vi "Set Point.vi"(8 "error in (no error)":errorcluster, 9 "Output #":i32=1, 10 "Set point":dbl, 11 "Cryo-Con Driver in":refnum<class "Cryo-Con Driver.lvclass">) -> (0 "error out":errorcluster, 3 "Cryo-Con Driver out":refnum<class "Cryo-Con Driver.lvclass">)   [LabVIEW 2021, in "Cryo-Con Driver.lvclass"]
uses:
  Cryo-Con Driver.lvclass
  C:/GitHub/NHMFL_Core/Libraries/Instruments/VISA Instrument/VISA Instrument.lvclass
  VISA Instrument/VISA Instrument.lvclass/VISA Instrument.ctl
  VISA Instrument/Read VISA resource.vi
  VISA Instrument/Write VISA resource.vi
  Cryo-Con Driver.lvclass/Cryo-Con Driver.ctl
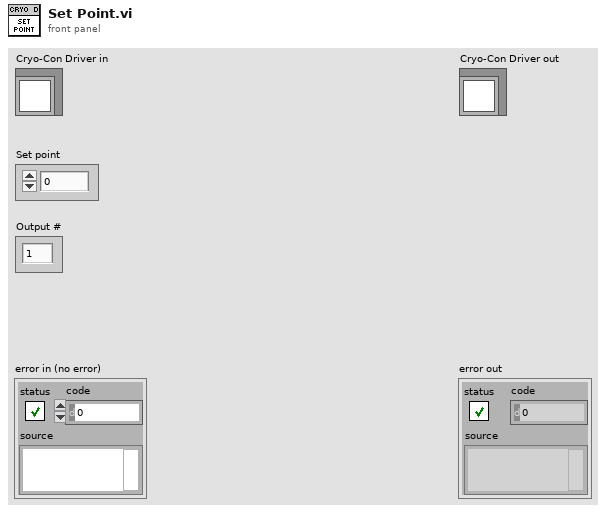
[diagram p1: front panel]
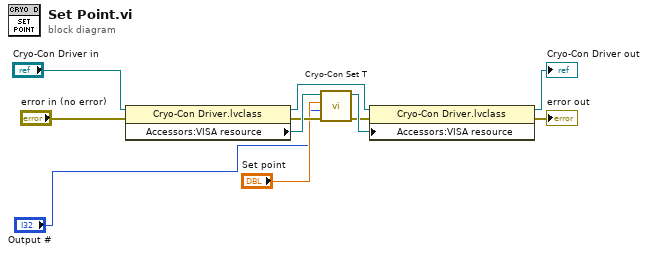
[diagram p0: block diagram]
diagram:
  n1 = property class="Cryo-Con Driver.lvclass"(reference="Cryo-Con Driver in", error in="error in (no error)") -> (reference out=w11:refnum<class "Cryo-Con Driver.lvclass">, error out=w6:errorcluster, "Accessors:VISA resource"=w9:refnum<visa-resource-name>)
  n2 = call "Cryo-Con Set T.vi"("error in (no error)"=w6, "Output #"="Output #", "Set T"="Set point", "VISA Resource Name"=w9) -> ("error out"=w7:errorcluster, "VISA Resource Name Out"=w8:refnum<visa-resource-name>)  [unwired: 6 in]
  n3 = property class="Cryo-Con Driver.lvclass"(reference=w11, error in=w7, "Accessors:VISA resource"=w8) -> (reference out=→"Cryo-Con Driver out":refnum<class "Cryo-Con Driver.lvclass">, error out=→"error out":errorcluster)
